vi "find row in string array.vi"(8 "error in (no error)":errorcluster, 9 "parameter name":string, 10 "limit values":string[][](array[string]), 11 "Simulated_CCD_Camera in":refnum<class "Simulated Camera.lvclass">) -> (0 "error out":errorcluster, 2 "row":string[](array[string]), 3 "Simulated_CCD_Camera out":refnum<class "Simulated Camera.lvclass">)   [LabVIEW 2018, in "Simulated Camera.lvclass"]
uses:
  Simulated Camera.lvclass
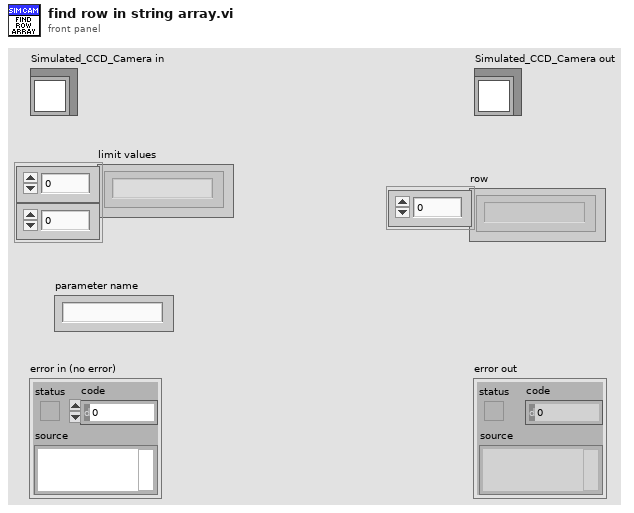
[diagram p1: front panel]
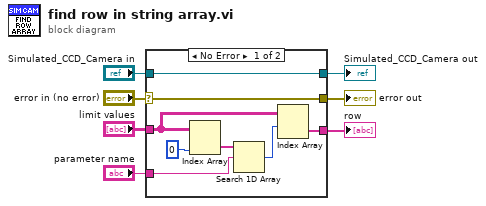
[diagram p0: block diagram]
diagram:
  n1 = case shown="No Error" "error in (no error)" {
    selector: "error in (no error)" -> [w14 w17]
    tunnel: [w14 w17] -> w6
    tunnel: [w15 w16] -> w4
    tunnel: "Simulated_CCD_Camera in" -> [w15 w16]
    tunnel: "limit values" -> [w9 _]
    tunnel: "parameter name" -> [w10 _]
    tunnel: [w8 _] -> w1
    frame No Error {
      n2 = Index Array(array=w9, index (col)=0 ("disabled index (col)")) -> (element=w11:string[])  [unwired: 1 in]
      n3 = Search 1D Array(1D array=w11, element=w10) -> (index of element=w12:i32)  [unwired: 1 in]
      n4 = Index Array(array=w9, index (row)=w12) -> (element=w8:string[])  [unwired: 1 in]
    }
    frame Error {
    }
  }
  "error out" <- w6
  "Simulated_CCD_Camera out" <- w4
  "row" <- w1
